vi "GMLAN DefinePIDByAddress.vi"(6 "MemorySize":u8, 7 "MemoryAddressLength":enum8{"Two", "Three", "Four"}(ring), 8 "error in (no error)":errorcluster, 9 "PIDAddress":u16, 10 "MemoryAddress":u32, 11 "diag ref in":T1) -> (0 "error out":errorcluster, 1 "success?":bool, 2 "data out":u8[](array[numeric]), 3 "diag ref out":T1)   [LabVIEW 2015, in "GMLAN.lvlib"]
uses:
  GMLAN.lvlib
  <vilib>/Automotive Diagnostic Command Set/Diagnostic Transport.llb/Diag Reference.ctl
  <vilib>/Automotive Diagnostic Command Set/Diagnostic Transport.llb/Transport Protocol Selector.ctl
  <vilib>/Automotive Diagnostic Command Set/Diagnostic Transport.llb/Diag CAN Frame Log.ctl
  <vilib>/addons/Automotive Diagnostic Command Set/NI_Automotive Diagnostic Command Set.lvlib
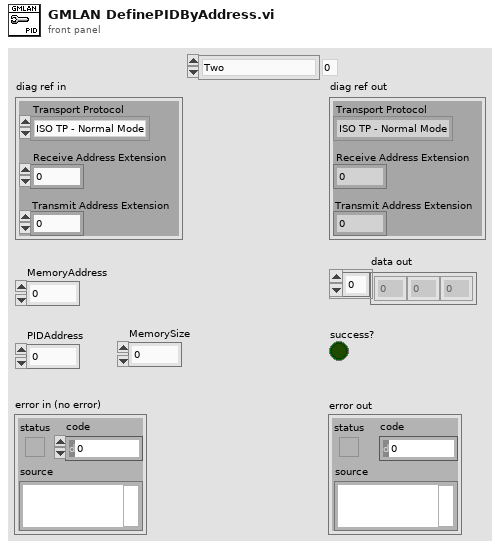
[diagram p1: front panel]
types:
  T1 = typedef "NI_Automotive Diagnostic Command Set.lvlib/Diag Reference.ctl" = cluster{"Diag CAN Handle":u32, "Transport Protocol":T2, "Receive Address Extension":u8, "Transmit Address Extension":u8, "Receive CAN Id":u32, "Transmit CAN Id":u32, "Diag CAN Queue":refnum<queue>, "Log Frames ?":bool, "My TP Address":u8, "Other TP Address":u8, "T1":u16, "T2":u16, "T3":u16, "T4":u16, "Tx SN":u8, "Block Size":u8, "Rx SN":u8, "VW TP Initialized?":bool, "Tx block no":u8, "baud rate":u32, "Interface":string, "Channel Diag CAN Handle":u32, "UDP Connection ID":refnum<k16>, "TCP Connection ID":refnum<k5>, "Target IP Addr":u32, "Source Address":u16, "Target Address":u16, "Send Header NACK?":bool, "DLL Handle":u32, "NAD":u8, "Time Stamp read first":dbl, "Time Stamp read last":dbl, "Time Stamp write first":dbl, "Time Stamp write last":dbl, "Time Stamp write":dbl, "Time Stamp read":dbl}
  T2 = typedef "NI_Automotive Diagnostic Command Set.lvlib/Transport Protocol Selector.ctl" = enum16{"ISO TP - Normal Mode", "ISO TP - Mixed Mode", "VW TP 2.0", "Diagnostics on IP", "ISO TP LIN"}
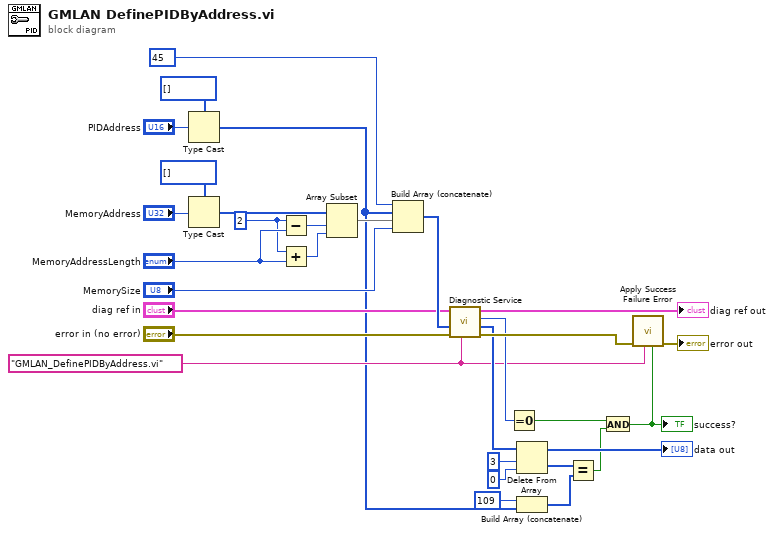
[diagram p0: block diagram]
diagram:
  w6 = 2 ("index")
  w14 = "GMLAN_DefinePIDByAddress.vi" ("error source")
  n1 = Type Cast(type=u8[] [], x="PIDAddress") -> (*(type *) &x=w1:u8[])
  n2 = Type Cast(type=u8[] [], x="MemoryAddress") -> (*(type *) &x=w9:u8[])
  n3 = Subtract(x=w6, y="MemoryAddressLength") -> (x-y=w7:i32)
  n4 = Add(x=w6, y="MemoryAddressLength") -> (x+y=w4:i32)
  n5 = Array Subset(array=w9, index=w7, length=w4) -> (w5:u8[])
  n6 = Build Array (concatenate)(u8 45 ("element"), w1, w5, "MemorySize") -> (w27:u8[])
  n7 = call <vilib>:"Diagnostic Service.vi"("error source"=w14, "error in (no error)"="error in (no error)", "data in"=w27, "diag ref in"="diag ref in") -> ("error out"=w29:errorcluster, "data out"=w22:u8[], "error code"=w26:u8, "diag ref out"=→"diag ref out":T1)  [unwired: 2 in, 2 out]
  n8 = Equal To 0?(x=w26) -> (x = 0?=w20:bool)
  n9 = Delete From Array(array=w22, length=3, index=0) -> (deleted portion=w21:u8[], array with subset deleted=→"data out":u8[])
  n10 = Build Array (concatenate)(u8 109 ("element"), w1) -> (w23:u8[])
  n11 = Equal?(x=w21, y=w23) -> (x = y?=w18:bool)
  n12 = And(x=w20, y=w18) -> (x .and. y?=w15:bool)
  "success?" <- w15
  n13 = call <vilib>:"Apply Success Failure Error.vi"("success code"=w15, "error source"=w14, "error in (no error)"=w29) -> ("error out"=→"error out":errorcluster)  [unwired: 8 out]
